vi "xyz_to_xy.vi"(2 "Position":cluster{"x":dbl, "y":dbl, "z":dbl}) -> (6 "Position (2D)":cluster{"x":dbl, "y":dbl}, 7 "z":dbl)   [LabVIEW 2010]
doc: "This VI splits a cluster of x,y,z into a cluster of x,y and a scalar z value"
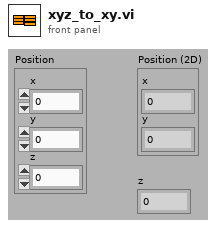
[diagram p1: front panel]
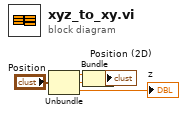
[diagram p0: block diagram]
diagram:
  n1 = Unbundle("Position") -> ("x"=w2:dbl, "y"=w1:dbl, "z"=→"z":dbl)
  n2 = Bundle("x"=w2, "y"=w1) -> (→"Position (2D)":cluster{"x":dbl, "y":dbl})  [unwired: 1 out]
